vi "ReadIOSettings.vi"   [LabVIEW 2020]
uses:
  global/SettingVariable.vi
  <vilib>/Utility/config.llb/Read Key (Boolean).vi
  <vilib>/Utility/config.llb/Read Key (String).vi
  <vilib>/Utility/config.llb/Read Key (I32).vi
  <vilib>/Utility/config.llb/Read Key (Double).vi
  <vilib>/Utility/config.llb/Read Key (U32).vi
  <vilib>/Utility/config.llb/Read Key (Path).vi
  <vilib>/Utility/config.llb/NI_LVConfig.lvlib
types:
  T1 = typedef "NI_LVConfig.lvlib/Config Data RefNum.ctl" = refnum<k1>
  T2 = cluster{"switch":bool, "voltage upper":i32, "voltage lower":i32, "physics upper":dbl, "physics lower":dbl, "input":u16, "log":bool}[]
  T3 = cluster{"switch":bool, "name":string, "voltage upper":i32, "voltage lower":i32, "physics upper":dbl, "physics lower":dbl, "scale":u16}[]
  T4 = cluster{"switch":bool, "name":string, "voltage upper":i32, "voltage lower":i32, "physics upper":dbl, "physics lower":dbl, "scale":u16}
  T5 = cluster{"switch":bool, "voltage upper":i32, "voltage lower":i32, "physics upper":dbl, "physics lower":dbl, "input":u16, "log":bool}
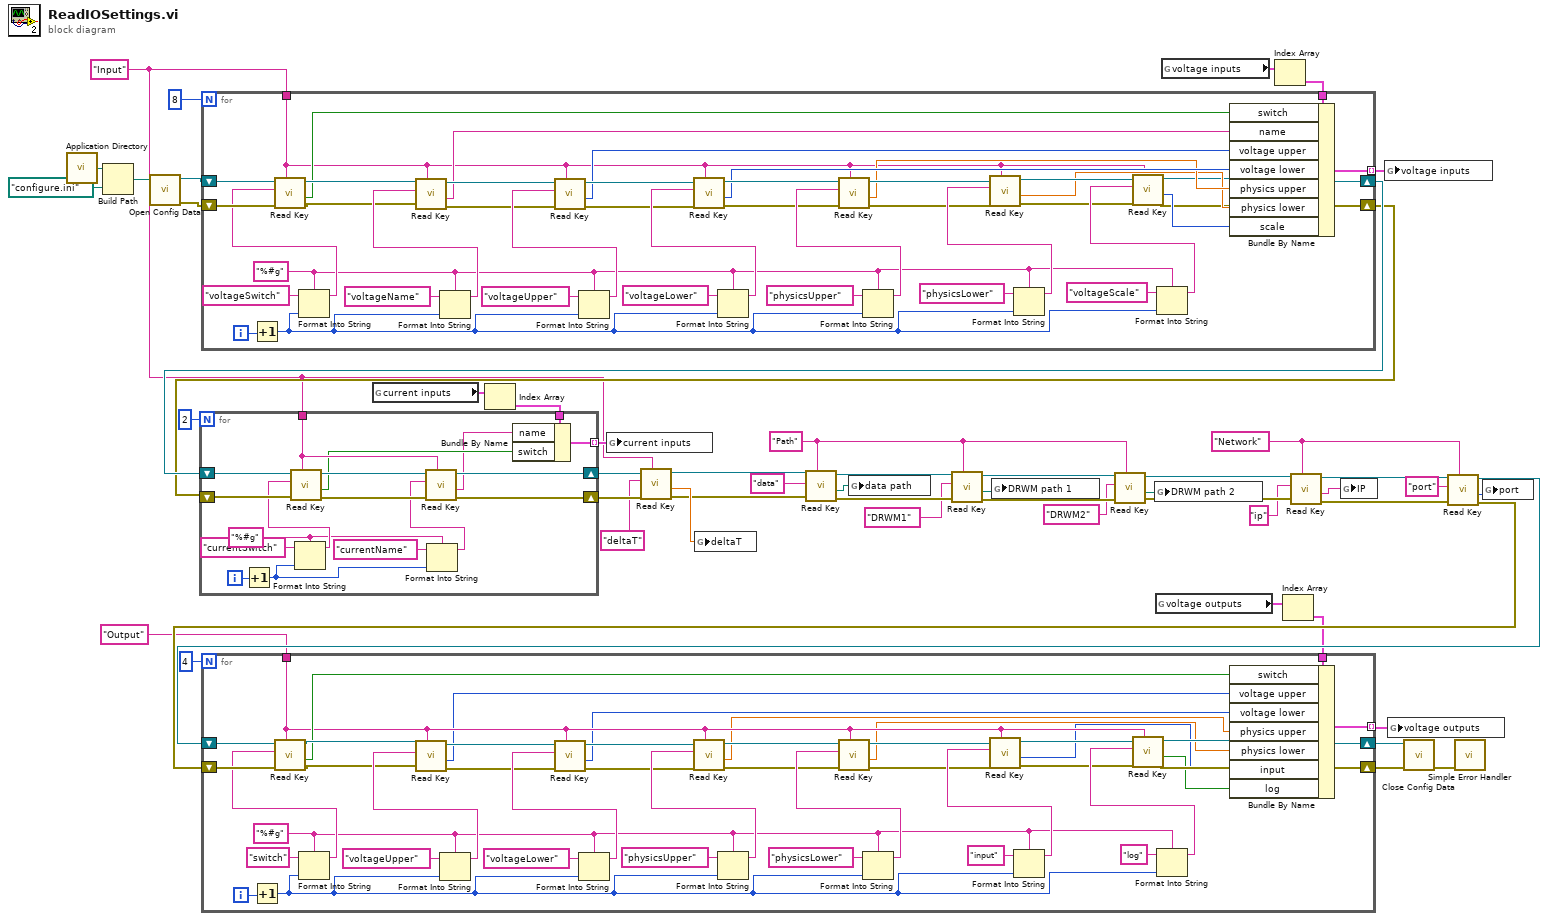
[diagram p0: block diagram]
diagram:
  w19 = "Network" ("section")
  w23 = "Path" ("section")
  w31 = "Input" ("section")
  n1 = call <vilib>:"Application Directory.vi"() -> ("Application Directory"=w52:path)
  n2 = Build Path(base path=w52, name or relative path=path "configure.ini") -> (appended path=w50:path)
  n3 = call <vilib>:"Open Config Data.vi"("configuration file path"=w50) -> ("error out"=w46:errorcluster, "refnum"=w47:T1)  [unwired: 8 in, 1 out]
  n4 = global read "SettingVariable.vi" "current inputs"() -> (w49:cluster{"name":string, "switch":bool}[])
  n5 = Index Array(array=w49) -> (element=w39:cluster{"name":string, "switch":bool})  [unwired: 1 in]
  n6 = global read "SettingVariable.vi" "voltage outputs"() -> (w5:T2)
  n7 = global read "SettingVariable.vi" "voltage inputs"() -> (w48:T3)
  n8 = Index Array(array=w48) -> (element=w45:T4)  [unwired: 1 in]
  n9 = for {
    N: 8 -> [_]
    tunnel: w31 -> [w56]
    tunnel: w45 -> [w66]
    tunnel: [w57] -> w44 mode=indexing
    shift-right: [w55] -> w41
    shift-left: w46 -> [w93]
    shift-right: [w54] -> w42
    shift-left: w47 -> [w94]
    i -> [w95]
    w53 = "%#g" ("format string")
    n10 = Increment(x=w95) -> (x+1=w64:i32)
    n11 = Format Into String(format string=w53, initial string="voltageSwitch", w64) -> (resulting string=w91:string)  [unwired: 1 in, 1 out]
    n12 = call-poly <vilib>:"Read Key.vi"("section"=w56, "error in (no error)"=w93, "key"=w91, "refnum"=w94) -> ("error out"=w87:errorcluster, "value"=w63:bool, "refnum out"=w88:T1)  [unwired: 4 in, 1 out]
    n13 = Format Into String(format string=w53, initial string="voltageName", w64) -> (resulting string=w90:string)  [unwired: 1 in, 1 out]
    n14 = call-poly <vilib>:"Read Key.vi"("section"=w56, "error in (no error)"=w87, "key"=w90, "refnum"=w88) -> ("error out"=w75:errorcluster, "value"=w62:string, "refnum out"=w76:T1)  [unwired: 4 in, 1 out]
    n15 = Format Into String(format string=w53, initial string="voltageUpper", w64) -> (resulting string=w85:string)  [unwired: 1 in, 1 out]
    n16 = call-poly <vilib>:"Read Key.vi"("section"=w56, "error in (no error)"=w75, "key"=w85, "refnum"=w76) -> ("error out"=w73:errorcluster, "value"=w61:i32, "refnum out"=w74:T1)  [unwired: 4 in, 1 out]
    n17 = Format Into String(format string=w53, initial string="voltageLower", w64) -> (resulting string=w84:string)  [unwired: 1 in, 1 out]
    n18 = call-poly <vilib>:"Read Key.vi"("section"=w56, "error in (no error)"=w73, "key"=w84, "refnum"=w74) -> ("error out"=w72:errorcluster, "value"=w60:i32, "refnum out"=w71:T1)  [unwired: 4 in, 1 out]
    n19 = Format Into String(format string=w53, initial string="physicsUpper", w64) -> (resulting string=w81:string)  [unwired: 1 in, 1 out]
    n20 = call-poly <vilib>:"Read Key.vi"("section"=w56, "error in (no error)"=w72, "key"=w81, "refnum"=w71) -> ("error out"=w69:errorcluster, "value"=w59:dbl, "refnum out"=w70:T1)  [unwired: 4 in, 1 out]
    n21 = Format Into String(format string=w53, initial string="physicsLower", w64) -> (resulting string=w80:string)  [unwired: 1 in, 1 out]
    n22 = call-poly <vilib>:"Read Key.vi"("section"=w56, "error in (no error)"=w69, "key"=w80, "refnum"=w70) -> ("error out"=w67:errorcluster, "value"=w58:dbl, "refnum out"=w68:T1)  [unwired: 4 in, 1 out]
    n23 = Format Into String(format string=w53, initial string="voltageScale", w64) -> (resulting string=w77:string)  [unwired: 1 in, 1 out]
    n24 = call-poly <vilib>:"Read Key.vi"("section"=w56, "error in (no error)"=w67, "key"=w77, "refnum"=w68) -> ("error out"=w55:errorcluster, "value"=w65:u32, "refnum out"=w54:T1)  [unwired: 4 in, 1 out]
    n25 = Bundle By Name(cluster=w66, "switch"=w63, "name"=w62, "voltage upper"=w61, "voltage lower"=w60, "physics upper"=w59, "physics lower"=w58, "scale"=w65) -> (w57:T4)
  }
  n26 = for {
    N: 2 -> [_]
    tunnel: w31 -> [w113]
    shift-right: [w105] -> w37
    shift-left: w42 -> [w110]
    shift-right: [w104] -> w36
    shift-left: w41 -> [w109]
    tunnel: w39 -> [w103]
    tunnel: [w100] -> w38 mode=indexing
    i -> [w108]
    w99 = "%#g" ("format string")
    n27 = Increment(x=w108) -> (x+1=w107:i32)
    n28 = Format Into String(format string=w99, initial string="currentSwitch", w107) -> (resulting string=w106:string)  [unwired: 1 in, 1 out]
    n29 = call-poly <vilib>:"Read Key.vi"("section"=w113, "error in (no error)"=w109, "key"=w106, "refnum"=w110) -> ("error out"=w112:errorcluster, "value"=w102:bool, "refnum out"=w111:T1)  [unwired: 4 in, 1 out]
    n30 = Format Into String(format string=w99, initial string="currentName", w107) -> (resulting string=w96:string)  [unwired: 1 in, 1 out]
    n31 = call-poly <vilib>:"Read Key.vi"("section"=w113, "error in (no error)"=w112, "key"=w96, "refnum"=w111) -> ("error out"=w104:errorcluster, "value"=w101:string, "refnum out"=w105:T1)  [unwired: 4 in, 1 out]
    n32 = Bundle By Name(cluster=w103, "name"=w101, "switch"=w102) -> (w100:cluster{"name":string, "switch":bool})
  }
  n33 = global write "SettingVariable.vi" "current inputs"(w38) -> ()
  n34 = call-poly <vilib>:"Read Key.vi"("section"=w31, "error in (no error)"=w36, "key"="deltaT", "refnum"=w37) -> ("error out"=w32:errorcluster, "value"=w34:dbl, "refnum out"=w33:T1)  [unwired: 4 in, 1 out]
  n35 = global write "SettingVariable.vi" "deltaT"(w34) -> ()
  n36 = call-poly <vilib>:"Read Key.vi"("section"=w23, "error in (no error)"=w32, "key"="data", "refnum"=w33) -> ("error out"=w27:errorcluster, "value"=w30:path, "refnum out"=w26:T1)  [unwired: 4 in, 1 out]
  n37 = global write "SettingVariable.vi" "data path"(w30) -> ()
  n38 = call-poly <vilib>:"Read Key.vi"("section"=w23, "error in (no error)"=w27, "key"="DRWM1", "refnum"=w26) -> ("error out"=w24:errorcluster, "value"=w29:path, "refnum out"=w25:T1)  [unwired: 4 in, 1 out]
  n39 = global write "SettingVariable.vi" "DRWM path 1"(w29) -> ()
  n40 = call-poly <vilib>:"Read Key.vi"("section"=w23, "error in (no error)"=w24, "key"="DRWM2", "refnum"=w25) -> ("error out"=w16:errorcluster, "value"=w28:path, "refnum out"=w17:T1)  [unwired: 4 in, 1 out]
  n41 = global write "SettingVariable.vi" "DRWM path 2"(w28) -> ()
  n42 = Index Array(array=w5) -> (element=w4:T5)  [unwired: 1 in]
  n43 = call-poly <vilib>:"Read Key.vi"("section"=w19, "error in (no error)"=w16, "key"="ip", "refnum"=w17) -> ("error out"=w15:errorcluster, "value"=w13:string, "refnum out"=w18:T1)  [unwired: 4 in, 1 out]
  n44 = global write "SettingVariable.vi" "IP"(w13) -> ()
  n45 = global write "SettingVariable.vi" "voltage inputs"(w44) -> ()
  n46 = call-poly <vilib>:"Read Key.vi"("section"=w19, "error in (no error)"=w15, "key"="port", "refnum"=w18) -> ("error out"=w6:errorcluster, "value"=w11:u32, "refnum out"=w7:T1)  [unwired: 4 in, 1 out]
  n47 = for {
    N: 4 -> [_]
    tunnel: "Output" ("section") -> [w123]
    tunnel: w4 -> [w127]
    tunnel: [w124] -> w1 mode=indexing
    shift-right: [w122] -> w8
    shift-left: w6 -> [w154]
    shift-right: [w121] -> w9
    shift-left: w7 -> [w155]
    i -> [w156]
    w120 = "%#g" ("format string")
    n48 = Increment(x=w156) -> (x+1=w126:i32)
    n49 = Format Into String(format string=w120, initial string="switch", w126) -> (resulting string=w152:string)  [unwired: 1 in, 1 out]
    n50 = call-poly <vilib>:"Read Key.vi"("section"=w123, "error in (no error)"=w154, "key"=w152, "refnum"=w155) -> ("error out"=w148:errorcluster, "value"=w125:bool, "refnum out"=w149:T1)  [unwired: 4 in, 1 out]
    n51 = Format Into String(format string=w120, initial string="voltageUpper", w126) -> (resulting string=w151:string)  [unwired: 1 in, 1 out]
    n52 = call-poly <vilib>:"Read Key.vi"("section"=w123, "error in (no error)"=w148, "key"=w151, "refnum"=w149) -> ("error out"=w136:errorcluster, "value"=w118:i32, "refnum out"=w137:T1)  [unwired: 4 in, 1 out]
    n53 = Format Into String(format string=w120, initial string="voltageLower", w126) -> (resulting string=w146:string)  [unwired: 1 in, 1 out]
    n54 = call-poly <vilib>:"Read Key.vi"("section"=w123, "error in (no error)"=w136, "key"=w146, "refnum"=w137) -> ("error out"=w134:errorcluster, "value"=w117:i32, "refnum out"=w135:T1)  [unwired: 4 in, 1 out]
    n55 = Format Into String(format string=w120, initial string="physicsUpper", w126) -> (resulting string=w145:string)  [unwired: 1 in, 1 out]
    n56 = call-poly <vilib>:"Read Key.vi"("section"=w123, "error in (no error)"=w134, "key"=w145, "refnum"=w135) -> ("error out"=w133:errorcluster, "value"=w116:dbl, "refnum out"=w132:T1)  [unwired: 4 in, 1 out]
    n57 = Format Into String(format string=w120, initial string="physicsLower", w126) -> (resulting string=w142:string)  [unwired: 1 in, 1 out]
    n58 = call-poly <vilib>:"Read Key.vi"("section"=w123, "error in (no error)"=w133, "key"=w142, "refnum"=w132) -> ("error out"=w130:errorcluster, "value"=w115:dbl, "refnum out"=w131:T1)  [unwired: 4 in, 1 out]
    n59 = Format Into String(format string=w120, initial string="input", w126) -> (resulting string=w141:string)  [unwired: 1 in, 1 out]
    n60 = call-poly <vilib>:"Read Key.vi"("section"=w123, "error in (no error)"=w130, "key"=w141, "refnum"=w131) -> ("error out"=w128:errorcluster, "value"=w114:u32, "refnum out"=w129:T1)  [unwired: 4 in, 1 out]
    n61 = Format Into String(format string=w120, initial string="log", w126) -> (resulting string=w138:string)  [unwired: 1 in, 1 out]
    n62 = call-poly <vilib>:"Read Key.vi"("section"=w123, "error in (no error)"=w128, "key"=w138, "refnum"=w129) -> ("error out"=w122:errorcluster, "value"=w119:bool, "refnum out"=w121:T1)  [unwired: 4 in, 1 out]
    n63 = Bundle By Name(cluster=w127, "switch"=w125, "voltage upper"=w118, "voltage lower"=w117, "physics upper"=w116, "physics lower"=w115, "input"=w114, "log"=w119) -> (w124:T5)
  }
  n64 = global write "SettingVariable.vi" "voltage outputs"(w1) -> ()
  n65 = call <vilib>:"Close Config Data.vi"("error in (no error)"=w8, "refnum"=w9) -> ("error out"=w10:errorcluster)  [unwired: 8 in, 1 out]
  n66 = call <vilib>:"Simple Error Handler.vi"("error in (no error)"=w10) -> ()  [unwired: 1 in, 8 out]
  n67 = global write "SettingVariable.vi" "port"(w11) -> ()
